vi "Compare Variable lists.vi"(8 "error in (no error)":errorcluster, 10 "Channel Arrays":T1, 11 "Variable List":refnum<class "ChannelVS.lvclass">[](array[class])) -> (0 "error out":errorcluster, 3 "Variable list compared":refnum<class "ChannelVS.lvclass">[](array[class]))   [LabVIEW 2017, in "Shared Variables CD 2.0 Configuration.lvlib" / "ChannelVS.lvclass"]
uses:
  ChannelVS.lvclass
  ChannelVS.lvclass/ChannelVS.ctl
  Read VeriSTAND Channel Info.vi
  Write VeriSTAND Channel Info.vi
  Public/Documents/National Instruments/NI VeriStand 2017/Custom Devices/Shared Variables CD 2.0/Data/Channel.lvlibp/Read Channel Info.vi
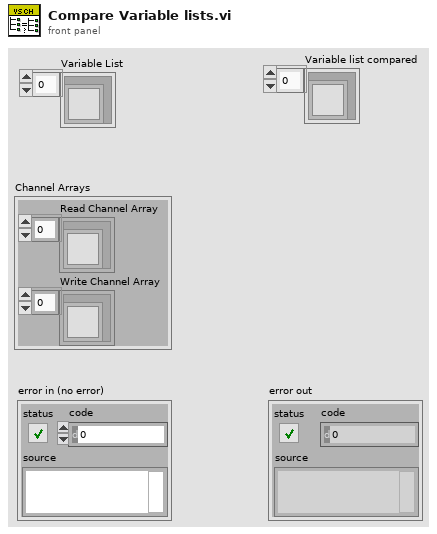
[diagram p1: front panel]
types:
  T1 = cluster{"Read Channel Array":refnum<class "ChannelVS.lvclass">[], "Write Channel Array":refnum<class "ChannelVS.lvclass">[]}
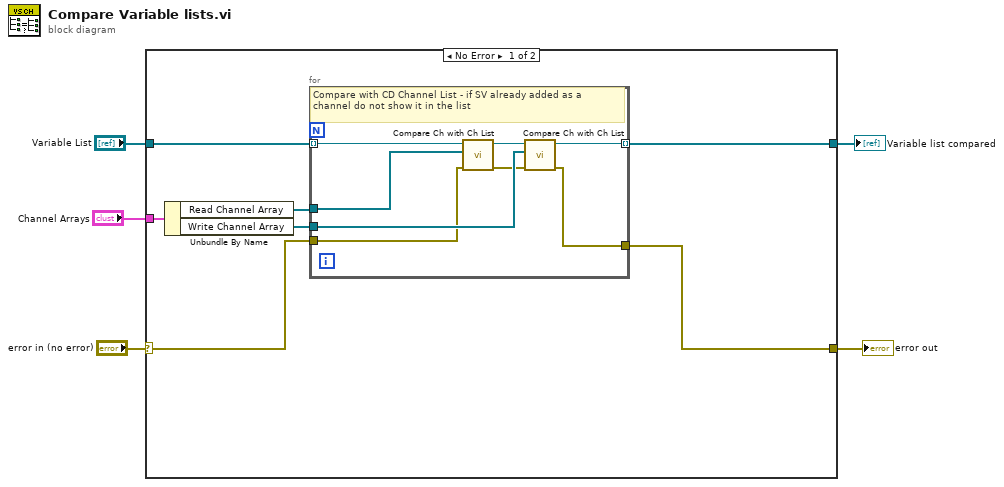
[diagram p0: block diagram]
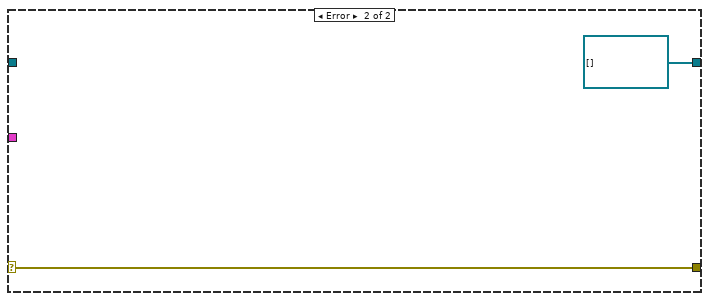
[diagram p2: hidden frame]
diagram:
  n1 = case shown="No Error" "error in (no error)" {
    selector: "error in (no error)" -> [w7 w22]
    tunnel: "Channel Arrays" -> [w10 _]
    tunnel: "Variable List" -> [w9 _]
    tunnel: [w6 w22] -> w3
    tunnel: [w8 refnum<class "ChannelVS.lvclass">[] []] -> w1
    frame No Error {
      n2 = Unbundle By Name(w10) -> ("Read Channel Array"=w11:refnum<class "ChannelVS.lvclass">[], "Write Channel Array"=w12:refnum<class "ChannelVS.lvclass">[])
      n3 = for {
        tunnel: w9 -> [w18] mode=indexing
        tunnel: w11 -> [w20]
        tunnel: [w17] -> w8 mode=indexing
        tunnel: w12 -> [w19]
        tunnel: w7 -> [w14]
        tunnel: [w13] -> w6
        # "Compare with CD Channel List - if SV already added as a channel do not show it in the list"
        n4 = call "Compare Ch with Ch List.vi"("error in (no error)"=w14, "Compare List"=w20, "Channel to compare"=w18) -> ("error out"=w15:errorcluster, "Channel out"=w16:refnum<class "ChannelVS.lvclass">)  [unwired: 7 in]
        n5 = call "Compare Ch with Ch List.vi"("error in (no error)"=w15, "Compare List"=w19, "Channel to compare"=w16) -> ("error out"=w13:errorcluster, "Channel out"=w17:refnum<class "ChannelVS.lvclass">)  [unwired: 7 in]
      }
    }
    frame Error {
    }
  }
  "Variable list compared" <- w1
  "error out" <- w3
